vi "UHR-Fleezers Control (host) - Lorentz v5.vi"() -> ()   [LabVIEW 2014] (continued)
          n904 = property on="Invert laser interlacing" class="Bool (strict)"("Val(Sgnl)"=w1399) -> ()  [unwired: 2 in, 2 out]
          n905 = property on="Laser interlacing mode" class="RadioBtnsControl (strict)"("Val(Sgnl)"=w1400) -> ()  [unwired: 2 in, 2 out]
        }
        frame #2 {
          w1402 = path "C:/Home/Bustamante Lab/Comstock-LabView-Link.udl" ("connection information")
          # "Database link changed by Ronen - not clear if it matter for the program."
          # "Initialize the database connection"
          n906 = disable-structure shown="Disabled" {
            disable-tunnel: [w1405 _] -> w1403
            disable-tunnel: w1402 -> [w1404 _]
            frame Disabled {
              n907 = call-poly <vilib>:"DB Tools Open Connection.vi"("connection information"=w1404) -> ("connection reference"=w1405:T24)  [unwired: 7 in, 1 out]
            }
            frame Enabled {
            }
          }
          "connection reference" <- w1403
          n908 = local write "connection reference"(w1403) -> ()
          n909 = local write "Database link"(w1402) -> ()
        }
        frame #3 {
          # "Load active calibration to fpga"
          n910 = local read "Base N trap periods"() -> (w1407:u32)
          n911 = local read "T1 Osc Enable"() -> (w1406:bool)
          n912 = property on="T1 Osc Enable" class="Bool (strict)"("Val(Sgnl)"=w1406) -> ()  [unwired: 2 in, 2 out]
          n913 = property on="Base N trap periods" class="DigNum (strict)"("Val(Sgnl)"=w1407) -> ()  [unwired: 2 in, 2 out]
        }
      }
    }
    frame #4 {
      # "Set FIFO size and run FPGA"
      n914 = local read "FPGA error out"() -> (w1409:errorcluster)
      n915 = xnode "Invoke Method"("FPGA VI Reference In"=w1410, "error in"=w1409, "Requested Depth"="Trap AI FIFO Depth") -> ("FPGA VI Reference Out"=w1414:T35, "error out"=w1415:errorcluster)  [unwired: 1 out]
      n916 = xnode "Invoke Method"("FPGA VI Reference In"=w1414, "error in"=w1415, "Requested Depth"="Trap Position FIFO Depth") -> ("FPGA VI Reference Out"=w1412:T35, "error out"=w1411:errorcluster)  [unwired: 1 out]
      n917 = xnode "Invoke Method"("FPGA VI Reference In"=w1412, "error in"=w1411) -> ("error out"=w1408:errorcluster)  [unwired: 1 in, 1 out]
      n918 = local write "FPGA error out"(w1408) -> ()
    }
    frame #5 {
      # "Adjust FPGA timing loop phases"
      n919 = flat-sequence "Initial FPGA Loop Relative Phase Adjustment" {
        tunnel: "Initial Phase Adjustment (AI1)" -> [w1449]
        tunnel: "Initial Phase Adjustment (GI)" -> [w1448]
        tunnel: "Initial Phase Adj. (MCL)" -> [w1447]
        tunnel: [w1450] -> w1434
        tunnel: [w1446] -> w1433
        tunnel: "Initial Phase Adjustment (APD Acq)" -> [w1445]
        tunnel: "Initial Phase Adjustment (APD 1 Gate)" -> [w1444]
        tunnel: "Initial Phase Adjustment (Green FB)" -> [w1443]
        tunnel: "Initial Phase Adjustment (GI) 2" -> [w1442]
        tunnel: "Initial Phase Adjustment (APD 2 Gate)" -> [w1441]
        tunnel: "Initial Phase Adjustment (RI)" -> [w1440]
        tunnel: "Initial Phase Adjustment (BI DO)" -> [w1439]
        tunnel: "Initial Phase Adjustment (BI AO)" -> [w1438]
        tunnel: "Initial Phase Adjustment (APD 3 Gate)" -> [w1437]
        tunnel: w1419 -> [w1436]
        tunnel: w1434 -> [w1452]
        tunnel: [w1453] -> w1432
        tunnel: w1433 -> [w1453]
        tunnel: [w1452] -> w1431
        tunnel: w1432 -> [w1457]
        tunnel: w1431 -> [w1456]
        tunnel: [w1454] -> w1418
        frame #0 {
          n920 = local read "FPGA error out"() -> (w1435:errorcluster)
          n921 = xnode "Read/Write Control"("FPGA VI Reference In"=w1436, "error in"=w1435, "Phase count adjustment"=w1449, "Phase count adjustment (GI)"=w1448, "Phase count adjustment (MCL)"=w1447, "Phase Count Adjustment (APD Acq)"=w1445, "Phase count adjustment (APD 1 Gate)"=w1444, "Phase count adjustment (APD 2 Gate)"=w1441, "Phase count adjustment (Green FB)"=w1443, "Phase count adjustment (GI) 2"=w1442, "Phase count adjustment (RI)"=w1440, "Phase count adjustment (BI AO)"=w1438, "Phase count adjustment (BI D)"=w1439, "Phase count adjustment (APD 3 Gate)"=w1437) -> ("FPGA VI Reference Out"=w1446:T35, "error out"=w1450:errorcluster)
        }
        frame #1 {
          n922 = Wait (ms)(milliseconds to wait=u32 100) -> ()  [unwired: 1 out]
        }
        frame #2 {
          w1455 = TRUE
          n923 = xnode "Read/Write Control"("FPGA VI Reference In"=w1457, "error in"=w1456, "+ phase"=w1455, "+ phase (GI)"=w1455, "+ phase (MCL)"=w1455, "+ phase (APD Acq)"=w1455, "+ phase (APD 1 Gate)"=w1455, "+ phase (APD 2 Gate)"=w1455, "+ phase (Green FB)"=w1455, "+ phase (GI) 2"=w1455, "+ phase (RI)"=w1455, "+ phase (BI AO)"=w1455, "+ phase (BI D)"=w1455, "+ phase (APD 3 Gate)"=w1455) -> ("error out"=w1454:errorcluster)  [unwired: 1 out]
        }
      }
      n924 = local write "FPGA error out"(w1418) -> ()
    }
    frame #6 {
      w1471 = 6.0  # clock mult.
      w1470 = 49152000.0  # TCXO frequ.
      w1475 = 6.0  # clock mult.
      w1476 = 49152000.0  # TCXO frequ.
      # "Added by ronen - definition of \nlimit frequencies when using dynamic feedback"
      # "Initialize trap RF synth board and set initial frequencies and amplitudes"
      n925 = local read "FPGA error out"() -> (w1485:errorcluster)
      n926 = call "Initialize RF boards - interlace 3.vi"("error in"=w1485, "FPGA VI Reference In"=w1486) -> ("error out"=w1487:errorcluster, "FPGA VI Reference Out"=w1507:T35)
      n927 = call "set RF board frequency - interlace.vi"("Board 2 Frequency Limits"=w1482, "Board 1 Frequency Limits"=w1463, "error in"=w1487, "FPGA VI Reference In"=w1507, "Board 2 Frequency 3 (MHz)"="BD 2 Frequency 3 (MHz)", "Board 1 Frequency 3 (MHz)"="BD 1 Frequency 3 (MHz)", "Board 2 Frequency 2 (MHz)"="BD 2 Frequency 2 (MHz)", "Board 2 Frequency 1 (MHz)"="BD 2 Frequency 1 (MHz)", "Board 1 Frequency 2 (MHz)"="BD 1 Frequency 2 (MHz)", "Board 1 Frequency 1  (MHz)"="BD 1 Frequency 1 (MHz)") -> ("error out"=w1490:errorcluster, "FPGA VI Reference Out"=w1462:T35)
      n928 = Unbundle By Name(w1463) -> ("Maximum"=w1473:dbl, "Minimum"=w1464:dbl)
      n929 = call "set RF board amplitude - interlace.vi"("Board 2 Amplitude Limits"=w1484, "Board 1 Amplitude Limits"=w1483, "error in"=w1490, "FPGA VI Reference In"=w1462, "Board 2 Amplitude 3 (%)"="BD 2 Amplitude 3 (%)", "Board 1 Amplitude 3 (%)"="BD 1 Amplitude 3 (%)", "Board 2 Amplitude 2 (%)"="BD 2 Amplitude 2 (%)", "Board 2 Amplitude 1 (%)"="BD 2 Amplitude 1 (%)", "Board 1 Amplitude 2 (%)"="BD 1 Amplitude 2 (%)", "Board 1 Amplitude 1 (%)"="BD 1 Amplitude 1 (%)") -> ("error out"=w1459:errorcluster)  [unwired: 1 out]
      n930 = Multiply(x=w1464, y=1000000.0) -> (x*y=w1468:dbl)
      n931 = Multiply(x=w1473, y=1000000.0) -> (x*y=w1478:dbl)
      n932 = Scale By Power Of 2(n=48, x=w1468) -> (x*2^n=w1466:dbl)
      n933 = Subtract(x="BD 1 Frequency 1 (MHz)", y="BD 1 Frequency 2 (MHz)") -> (x-y=w1497:dbl)
      n934 = Subtract(x="BD 2 Frequency 1 (MHz)", y="BD 2 Frequency 2 (MHz)") -> (x-y=w1498:dbl)
      n935 = Scale By Power Of 2(n=48, x=w1478) -> (x*2^n=w1480:dbl)
      n936 = Multiply(x=w1470, y=w1471) -> (x*y=w1472:dbl)
      n937 = Multiply(x=w1476, y=w1475) -> (x*y=w1474:dbl)
      n938 = Square(x=w1498) -> (x^2=w1500:dbl)
      n939 = Square(x=w1497) -> (x^2=w1499:dbl)
      n940 = Divide(x=w1466, y=w1472) -> (x/y=w1467:dbl)
      n941 = Divide(x=w1480, y=w1474) -> (x/y=w1479:dbl)
      n942 = Add(x=w1499, y=w1500) -> (x+y=w1501:dbl)
      n943 = To Unsigned Quad Integer(1:w1467) -> (0:w1460:u64)
      n944 = To Unsigned Quad Integer(1:w1479) -> (0:w1461:u64)
      n945 = Square Root(x=w1501) -> (sqrt(x)=w1502:dbl)
      n946 = local write "Trap Delta (MHz)"(w1502) -> ()
      n947 = xnode "Read/Write Control"("FPGA VI Reference In"=w1462, "error in"=w1459, "FB Max Frequency"=w1461, "FB Min frequency"=w1460) -> ("error out"=w1458:errorcluster)  [unwired: 1 out]
      n948 = local write "FPGA error out"(w1458) -> ()
    }
    frame #7 {
      n949 = local read "FPGA error out"() -> (w1509:errorcluster)
      n950 = flat-sequence {
        tunnel: [w1523] -> w1514
        tunnel: [w1522] -> w1513
        tunnel: w1510 -> [w1516]
        tunnel: w1509 -> [w1515]
        tunnel: [w1527] -> w1512
        tunnel: w1514 -> [w1527]
        tunnel: [w1526] -> w1511
        tunnel: w1513 -> [w1526]
        tunnel: w1512 -> [w1535]
        tunnel: w1511 -> [w1534]
        tunnel: [w1529] -> w1508
        frame #0 {
          n951 = xnode "Read/Write Control"("FPGA VI Reference In"=w1516, "error in"=w1515, "Direct RF Box  Communication"=FALSE) -> ("FPGA VI Reference Out"=w1523:T35, "error out"=w1522:errorcluster)
          n952 = local read "Trap 1 (ON/OFF)"() -> (w1517:bool)
          n953 = local write "Saving..."(FALSE ("Saving Data")) -> ()
          n954 = local write "Stop All"(FALSE ("Stop All")) -> ()
          n955 = local write "Index"(1.0 ("Index")) -> ()
          n956 = property on="Trap 1 ON" class="Bool (strict)"("Value"=w1517) -> ()  [unwired: 2 in, 2 out]
          "Manipulating Trap" <- FALSE ("Manipulating Trap")
        }
        frame #1 {
          n957 = local read "Trap 2 (ON/OFF)"() -> (w1525:bool)
          n958 = Wait (ms)(milliseconds to wait=u32 10) -> ()  [unwired: 1 out]
          n959 = property on="Trap 2 ON" class="Bool (strict)"("Val(Sgnl)"=w1525) -> ()  [unwired: 2 in, 2 out]
        }
        frame #2 {
          n960 = local read "Scan Range (nm)"() -> (w1530:dbl)
          n961 = xnode "Read/Write Control"("FPGA VI Reference In"=w1535, "error in"=w1534, "FPGA Controls  RF Box"=TRUE ("Direct RF Box  Communication")) -> ("error out"=w1529:errorcluster)  [unwired: 1 out]
          n962 = call "Update messages.vi"("Message to add"="UHR-Fleezers ready.", "Old message string"="") -> ("New message string"=w1533:string)
          n963 = local write "Messages"(w1533) -> ()
          n964 = property on="Scan Range (nm)" class="DigNum (strict)"("Val(Sgnl)"=w1530) -> ()  [unwired: 2 in, 2 out]
        }
      }
      n965 = local write "FPGA error out"(w1508) -> ()
    }
    frame #8 {
      w1542 = u32 0
      w1548 = cluster{u32, u32} {16777238, 16777238}
      w1543 = 0.0
      n966 = control-ref of="Piezo trap cursor control"() -> (w1544:refnum<vi>)
      n967 = property class="XYGraph (strict)"(reference=w1544, "XScale.Maximum"=10.0, "XScale.Minimum"=w1543, "YScale.Maximum"=w1543, "YScale.Minimum"=-10.0, "Plot Area Colors"=w1548, "Frame Color"=u32 9868950, "XScale.GridColors"=w1548, "YScale.GridColors"=w1548, "Cursor.Cursor Color"=u32 16711680, "Active Cursor"=w1542, "Cursor.CursorMode"=w1542) -> ()  [unwired: 1 in, 2 out]
      n968 = call "hamilton_controller.vi"("VISA resource name in"="Visa resource for valves", "action"=T41."CONNECT") -> ("error out"=w1541:errorcluster, "VISA resource name out"=w1538:refnum<visa-resource-name>)  [unwired: 8 in]
      n969 = call "hamilton_controller.vi"("VISA resource name in"=w1538, "error in"=w1541, "action"=T41."INITIALIZE VALVES") -> ("error out"=w1550:errorcluster)  [unwired: 7 in, 1 out]
    }
    frame #9 {
      # "Wait 5 s for all the event loops still being executed to finish."
      n970 = Wait (ms)(milliseconds to wait=u32 5000) -> ()  [unwired: 1 out]
      n971 = local read "FPGA error out"() -> (w1552:errorcluster)
    }
  }
  n972 = node-c288() -> (w30:T36)  [unwired: 4 out]
  n973 = disable-structure shown="Disabled" {
    frame Disabled {
      n974 = while "Duncan's play event loop" {
        stop <- w1556 stop-if-true
        n975 = Create User Event(user event datatype=TRUE ("Boolean")) -> (user event=w1557:refnum<user-event>)  [unwired: 1 in, 1 out]
        n976 = Create User Event(user event datatype=TRUE ("Boolean")) -> (user event=w1563:refnum<user-event>)  [unwired: 1 in, 1 out]
        n977 = global write "Global for fluorescence simulation mean (30 samples), (power series).vi" "Red Signal"(w1557) -> ()
        n978 = global write "Global for fluorescence simulation mean (30 samples), (power series).vi" "Green Signal"(w1563) -> ()
        n979 = register-events(w1563, w1557) -> (reference out=w1562:refnum<event-registration>)  [unwired: 2 in, 1 out]
        n980 = event shown="[1] \"Start assembly line\": Value Change" {
          selector: w1562 -> [_ _ _ _]
          dyn-events: _ -> [_ _ _ _]
          timeout: 100 -> [_ _ _ _]
          event Timeout {
            n981 = event-data() -> ()  [unwired: 1 in, 2 out]
          }
          event "Start assembly line": Value Change {
            n982 = event-data() -> ("OldVal"=w1565:bool)  [unwired: 1 in, 4 out]
            n983 = case shown="True" w1565 {
              selector: w1565 -> [_ w1566]
              frame False {
              }
              frame True {
                n984 = property on="Move to Position 3" class="Bool"("Val(Sgnl)"=w1566) -> ()  [unwired: 2 in, 2 out]
                n985 = case shown="1" "Numeric" {
                  frame 0, Default {
                  }
                  frame 1 {
                    n986 = property on="Green Laser ON" class="Bool (strict)"("Val(Sgnl)"=TRUE ("Value (Signaling)")) -> ()  [unwired: 2 in, 2 out]
                  }
                  frame 2 {
                    n987 = property on="Red Laser ON" class="Bool (strict)"("Val(Sgnl)"=TRUE) -> ()  [unwired: 2 in, 2 out]
                  }
                }
              }
            }
          }
          event User Event {
            n988 = event-data() -> ("Boolean"=w1570:bool)  [unwired: 1 in, 3 out]
            "Green Fluorophore" <- w1570
            n989 = property on="Start assembly line" class="Bool"("Val(Sgnl)"=w1570) -> ()  [unwired: 2 in, 2 out]
          }
          event User Event {
            n990 = event-data() -> ("Boolean"=w1571:bool)  [unwired: 1 in, 3 out]
            "Red Fluorophore" <- w1571
            n991 = property on="Start assembly line" class="Bool"("Val(Sgnl)"=w1571) -> ()  [unwired: 2 in, 2 out]
          }
        }
        n992 = property on="Get Fluorophore" class="Bool (strict)"("Val(Sgnl)"="Get Fluorophore") -> ()  [unwired: 2 in, 2 out]
        n993 = Wait (ms)(milliseconds to wait=u32 100) -> ()  [unwired: 1 out]
        n994 = local read "Stop All"() -> (w1555:bool)
        n995 = Or(x=w1555, y="stop") -> (x .or. y?=w1556:bool)
      }
    }
    frame Enabled {
    }
  }
  n996 = timed-loop "Rough control of MCL mirror stage (debugging)" {
    tunnel: [w1574] -> w71
    timing: w30 -> [_]
    timing-out: [_] -> w29
    tunnel: w21 -> [w1572]
    stop <- w1574 stop-if-true
    n997 = node-c288() -> ()  [unwired: 2 out]
    n998 = case shown="1" "MCL Mode" {
      tunnel: w1572 -> [_ w1577 w1624]
      frame 0, Default {
      }
      frame 1 {
        n999 = node-c288() -> (w1579:T36)  [unwired: 4 out]
        n1000 = timed-loop "Oscillate MCL mirror" {
          timing: w1579 -> [_]
          timing-out: [_] -> w1578
          tunnel: w1577 -> [w1580]
          i -> [w1618]
          stop <- w1581 stop-if-true
          n1001 = node-c288() -> (w1617:i64)  [unwired: 1 out]
          n1002 = Multiply(x="AO1", y=32767.0) -> (x*y=w1613:dbl)
          n1003 = Multiply(x="AO2", y=32767.0) -> (x*y=w1608:dbl)
          n1004 = Divide(x=w1613, y=10.0) -> (x/y=w1614:dbl)
          n1005 = Divide(x=w1608, y=10.0) -> (x/y=w1609:dbl)
          n1006 = To Word Integer(number=w1614) -> (16bit integer=w1606:i16)
          n1007 = To Word Integer(number=w1609) -> (16bit integer=w1605:i16)
          n1008 = Divide(x=w1617, y=i64 1000) -> (x/y=w1588:dbl)
          n1009 = Multiply(x=w1588, y=w1618) -> (x*y=w1599:dbl)
          n1010 = Multiply(x="Osc. freq. (Hz) 2", y=6.283185307179586) -> (x*y=w1600:dbl)
          n1011 = Multiply(x=w1600, y=w1599) -> (x*y=w1598:dbl)
          n1012 = Sine(x=w1598) -> (sin(x)=w1597:dbl)
          n1013 = Multiply(x=w1597, y="Osc. amp. (V)") -> (x*y=w1595:dbl)
          n1014 = Add(x=w1595, y="Osc. center (V)") -> (x+y=w1593:dbl)
          n1015 = Divide(x=w1593, y=10.0) -> (x/y=w1591:dbl)
          n1016 = Multiply(x=w1591, y=32767.0) -> (x*y=w1586:dbl)
          n1017 = Select(t=w1586, s="Scan axis", f=w1606) -> (s? t:f=w1604:dbl)
          n1018 = Select(t=w1605, s="Scan axis", f=w1586) -> (s? t:f=w1603:dbl)
          n1019 = local read "MCL Mode"() -> (w1585:u16)
          n1020 = Not Equal?(x=w1585, y=u16 1) -> (x != y?=w1582:bool)
          n1021 = local read "Stop All"() -> (w1583:bool)
          n1022 = xnode "Read/Write Control"("FPGA VI Reference In"=w1580, "AO1"=w1604, "AO2"=w1603) -> ()  [unwired: 1 in, 2 out]
          n1023 = Compound Arithmetic op=OR(w1583, w1582) -> (w1581:bool)
          n1024 = node-c288() -> ()  [unwired: 2 out]
        }
        n1025 = node-c288(w1578) -> ()  [unwired: 1 out]
      }
      frame 2 {
        n1026 = case shown="True" "Start Scan" {
          tunnel: w1624 -> [_ w1626]
          frame False {
          }
          frame True {
            n1027 = Subtract(x="End (V)", y="Begin (V)") -> (x-y=w1633:dbl)
            n1028 = Decrement(x="N Points") -> (x-1=w1632:dbl)
            n1029 = Divide(x=w1633, y=w1632) -> (x/y=w1630:dbl)
            n1030 = for {
              N: "N Points" -> [_]
              tunnel: "Begin (V)" -> [w1649]
              tunnel: [w1641] -> w1636 mode=indexing
              tunnel: w1630 -> [w1640]
              tunnel: [w1638] -> w1629 mode=indexing
              tunnel: w1626 -> [w1637]
              i -> [w1648]
              n1031 = Multiply(x=w1640, y=w1648) -> (x*y=w1647:dbl)
              n1032 = Add(x=w1649, y=w1647) -> (x+y=w1644:dbl)
              n1033 = local read "Scan axis"() -> (w1639:bool)
              n1034 = local read "AO1"() -> (w1646:dbl)
              n1035 = local read "AO2"() -> (w1645:dbl)
              n1036 = Select(t=w1644, s=w1639, f=w1646) -> (s? t:f=w1643:dbl)
              n1037 = Select(t=w1645, s=w1639, f=w1644) -> (s? t:f=w1642:dbl)
              n1038 = flat-sequence {
                tunnel: w1643 -> [w1653]
                tunnel: w1642 -> [w1652]
                tunnel: w1637 -> [w1650]
                tunnel: [w1663] -> w1641
                tunnel: [w1662] -> w1638
                frame #0 {
                  w1656 = 10.0 ("y")
                  w1651 = 32767.0 ("y")
                  n1039 = Multiply(x=w1653, y=w1651) -> (x*y=w1659:dbl)
                  n1040 = Multiply(x=w1652, y=w1651) -> (x*y=w1657:dbl)
                  n1041 = Divide(x=w1659, y=w1656) -> (x/y=w1660:dbl)
                  n1042 = Divide(x=w1657, y=w1656) -> (x/y=w1658:dbl)
                  n1043 = To Word Integer(number=w1660) -> (16bit integer=w1654:i16)
                  n1044 = To Word Integer(number=w1658) -> (16bit integer=w1655:i16)
                  n1045 = xnode "Read/Write Control"("FPGA VI Reference In"=w1650, "AO1"=w1654, "AO2"=w1655) -> ()  [unwired: 1 in, 2 out]
                }
                frame #1 {
                  n1046 = Wait (ms)(milliseconds to wait="DAQ Delay (ms)") -> ()  [unwired: 1 out]
                }
                frame #2 {
                  n1047 = local read "Slow mean"() -> (w1663:dbl)
                  n1048 = local read "Sigma"() -> (w1662:dbl)
                }
              }
            }
            n1049 = Bundle("Begin (V)"="Begin (V)", w1630, w1636) -> (→"MCL Scan":cluster{"Begin (V)":dbl, dbl, dbl[]})  [unwired: 1 out]
            n1050 = Bundle("Begin (V)"="Begin (V)", w1630, w1629) -> (→"MCL Scan 2":cluster{"Begin (V)":dbl, dbl, dbl[]})  [unwired: 1 out]
          }
        }
      }
    }
    n1051 = local read "Stop All"() -> (w1574:bool)
    n1052 = node-c288() -> ()  [unwired: 2 out]
  }
  n1053 = node-c288(2 ("Processor")) -> (w62:T36)  [unwired: 3 out]
  n1054 = timed-loop "Basic control parameters (all FPGA settings, other basic controls)" {
    shift-right: [w1671] -> _
    shift-left: errorcluster {"status"=FALSE, "code"=0, "source"=""} ("error out") -> [_]
    tunnel: [w1670] -> _
    timing: w62 -> [_]
    timing-out: [_] -> w61
    tunnel: w43 -> [w1669]
    tunnel: w39 -> [w1668]
    tunnel: w38 -> [w1667]
    tunnel: w37 -> [w1666]
    tunnel: w36 -> [w1665]
    tunnel: w21 -> [w1664]
    stop <- w1670 stop-if-true
    n1055 = node-c288() -> ()  [unwired: 2 out]
    n1056 = event shown="[0] \"AI Count (ticks)\", \"Sets to FIFO (Traps)\", \"Save ave N\", \"FPGA Ave.\", \"# Samples/channel\", \"N sets to save\": Value Change" {
      selector: _ -> [_ _ _ _ _ _ _ _ _ _ _ _ _ _ _ _ _ _ _ _ _ _ _ _ _ _ _ _ _ _ _ _ _ _ _ _ _ _ _ _ _ _ _ _ _ _ _ _ _ _ _ _ _ _ _ _ _ _ _ _ _ _ _ _ _ _ _ _ _ _ _ _ _ _ _ _ _ _ _ _ _ _ _ _ _ _]
      dyn-events: _ -> [_ _ _ _ _ _ _ _ _ _ _ _ _ _ _ _ _ _ _ _ _ _ _ _ _ _ _ _ _ _ _ _ _ _ _ _ _ _ _ _ _ _ _ _ _ _ _ _ _ _ _ _ _ _ _ _ _ _ _ _ _ _ _ _ _ _ _ _ _ _ _ _ _ _ _ _ _ _ _ _ _ _ _ _ _ _]
      timeout: _ -> [_ _ _ _ _ _ _ _ _ _ _ _ _ _ _ _ _ _ _ _ _ _ _ _ _ _ _ _ _ _ _ _ _ _ _ _ _ _ _ _ _ _ _ _ _ _ _ _ _ _ _ _ _ _ _ _ _ _ _ _ _ _ _ _ _ _ _ _ _ _ _ _ _ _ _ _ _ _ _ _ _ _ _ _ _ _]
      tunnel: [w1711 _ _ _ w1738 _ _ _ _ _ _ _ w1844 _ _ w1931 w1933 w1940 w1942 w2012 _ w2054 w2080 w2108 w2133 w2160 w2186 w2215 _ w2220 w2314 w2318 w2355 _ w2418 w2421 w2424 w2434 w2437 _ w2444 _ _ _ _ _ _ _ _ _ _ _ _ _ _ _ _ _ _ _ w2939 _ _ _ _ w2976 _ _ _ _ _ _ _ _ _ _ _ _ _ _ _ _ _ _ _ _] -> w1671
      tunnel: [_ _ _ _ _ _ _ _ _ _ w1823 _ _ _ _ _ _ _ _ _ _ _ _ _ _ _ _ _ _ _ _ _ _ _ _ _ _ _ _ _ _ _ _ _ _ _ _ _ _ _ _ _ _ _ _ _ _ _ _ _ _ _ _ _ _ _ _ _ _ _ _ _ _ _ _ _ _ _ _ _ _ _ _ _ _ _] -> w1670
      tunnel: [_ _ _ _ _ _ _ _ "Round T1 X" _ _ _ _ _ _ _ _ _ _ _ _ _ _ _ _ _ _ _ _ _ _ _ _ _ _ _ _ _ _ _ _ _ _ _ _ _ _ _ _ _ _ _ _ _ _ _ _ _ _ _ _ _ _ _ _ _ _ _ _ _ _ _ _ _ _ _ _ _ _ _ _ _ _ _ _ _] -> _
      tunnel: [_ _ _ "Adjust Scale\nto Mean" _ _ _ _ _ _ _ _ _ _ _ _ _ _ _ _ _ _ _ _ _ _ _ _ _ "Test ttrig" _ _ _ _ _ _ _ _ _ _ _ _ _ _ _ _ _ _ _ _ w2686 w2750 w2797 w2846 _ _ _ _ _ _ _ _ _ _ _ _ _ _ _ _ _ _ _ _ _ _ _ _ _ _ _ _ _ _ _ _] -> _
      tunnel: [_ _ _ _ _ _ _ _ _ "Round T2 X" _ "Delayed Interlace Start" _ _ _ _ _ _ _ _ _ _ _ _ _ _ _ _ _ _ _ _ _ _ _ _ _ _ _ _ _ _ _ _ _ _ _ _ _ _ _ _ _ _ _ _ _ _ _ _ _ _ _ _ _ _ _ _ _ _ _ _ _ _ _ _ _ _ _ _ _ _ _ _ _ _] -> _
      tunnel: w1669 -> [_ _ _ _ _ _ _ _ _ _ _ _ _ _ _ _ _ _ _ _ _ _ _ _ _ _ _ _ _ _ _ _ _ _ _ _ _ _ _ _ _ _ _ _ _ _ w2656 w2664 w2671 w2677 w2685 _ _ w2845 _ _ _ _ _ _ _ _ _ _ _ _ _ _ _ _ _ _ _ _ _ _ _ _ _ _ _ _ _ _ _ _]
      tunnel: w1668 -> [_ _ _ _ _ _ _ _ _ _ _ _ _ _ _ _ _ _ _ _ _ _ _ _ _ _ _ _ _ _ _ _ _ _ _ _ _ _ _ _ _ _ _ _ w2543 _ _ _ _ _ _ w2749 _ _ w2852 _ w2864 _ w2880 _ _ _ _ _ _ _ _ _ _ _ _ _ _ _ _ _ _ _ _ _ _ _ _ _ _ _]
      tunnel: w1667 -> [_ _ _ _ _ _ _ _ _ _ _ _ _ _ _ _ _ _ _ _ _ _ _ _ _ _ _ _ _ _ _ _ _ _ _ _ _ _ _ _ _ _ _ _ _ _ _ _ _ _ _ _ _ _ _ _ _ _ _ _ _ _ _ _ _ _ _ _ _ _ _ _ _ _ _ _ _ _ _ _ _ _ _ _ _ _]
      tunnel: w1666 -> [_ _ _ _ _ _ _ _ _ _ _ _ _ _ _ _ _ _ _ _ _ _ _ _ _ _ _ _ _ _ _ _ _ _ _ _ _ _ _ _ _ w2455 _ _ _ _ _ _ _ _ _ _ w2796 _ _ w2858 _ w2872 _ w2906 _ _ _ _ _ _ _ _ _ _ _ _ _ _ _ _ _ _ _ _ _ _ _ _ _ _]
      tunnel: w1665 -> [_ _ _ _ _ _ _ _ _ _ _ _ _ _ _ _ _ _ _ _ _ _ _ _ _ _ _ _ _ _ _ _ _ _ _ _ _ _ _ _ _ _ _ _ _ _ _ _ _ _ _ _ _ _ _ _ _ _ _ _ _ _ _ _ _ _ _ _ _ _ _ _ _ _ _ _ _ _ _ _ _ _ _ _ _ _]
      tunnel: w1664 -> [w1674 _ _ _ w1737 _ w1763 _ _ _ _ _ w1835 _ _ w1915 w1932 w1939 w1941 w1977 _ w2043 w2078 w2090 w2115 w2143 w2163 w2191 w2216 w2218 w2222 w2315 w2319 _ w2415 w2419 w2422 w2432 w2435 _ w2443 _ _ _ _ _ _ _ _ _ _ _ _ _ _ _ _ _ _ _ w2932 _ w2953 _ w2960 w2975 _ w2982 w3009 w3016 w3032 w3040 _ w3051 _ w3095 _ _ w3149 w3180 w3184 w3192 _ w3256 w3266 w3285]
      tunnel: [_ _ _ _ _ _ _ _ _ _ w1822 _ _ _ _ _ _ _ _ _ _ _ _ _ _ _ _ _ _ _ _ _ _ _ _ _ _ _ _ _ _ _ w2535 w2539 _ _ _ _ _ _ _ _ _ _ _ _ _ _ _ _ _ _ _ _ _ _ _ _ _ _ _ _ _ _ _ _ _ _ _ _ _ _ _ _ _ _] -> _
      event "AI Count (ticks)", "Sets to FIFO (Traps)", "Save ave N", "FPGA Ave.", "# Samples/channel", "N sets to save": Value Change {
        # "RG 18-01-16 Increased amount of elements to read for trap position, to add x and y for piezo trap"
        # "So that if 'Save ave N' is updated, the AOD scanning code updates too."
        n1057 = event-data() -> ()  [unwired: 6 out]
        n1058 = local read "AI Count (ticks)"() -> (w1695:u16)
        n1059 = Divide(x=40000000.0, y=w1695) -> (x/y=w1687:dbl)
        "AI rate (Hz)" <- w1687
        "Ave. Rate (Hz)" <- w1687
        n1060 = Reciprocal(x=w1687) -> (1/x=→"Ave. Period (s)":dbl)
        n1061 = Unbundle By Name("Sets to FIFO (Traps)") -> ("Set 1"=w1678:bool, "Set 2"=w1677:bool, "Set 3"=w1676:bool)
        n1062 = Divide(x=w1687, y="N Acq Sets (Traps + Fl.)") -> (x/y=w1708:dbl)
        "Data Rate (Hz)" <- w1708
        n1063 = Reciprocal(x=w1708) -> (1/x=→"Data Period (s)":dbl)
        n1064 = Boolean To (0,1)(Boolean="Sets to FIFO (Traps)") -> (0, 1=w1703:cluster{"Set 1":i16, "Set 2":i16, "Set 3":i16})
        n1065 = xnode "Read/Write Control"("FPGA VI Reference In"=w1674, "ai count"=w1695, "Set 1"=w1678, "Set 2"=w1677, "Set 3"=w1676, "N of AI1 Int Acq Sets"="N Acq Sets (Traps + Fl.)") -> ("error out"=w1711:errorcluster)  [unwired: 1 in, 1 out]
        n1066 = Cluster To Array(cluster=w1703) -> (array=w1702:i16[])
        n1067 = local read "Save ave N"() -> (w1707:dbl)
        n1068 = To Unsigned Long Integer(number=w1702) -> (unsigned 32bit integer=w1684:u32[])
        n1069 = local read "Scan steps (AOD)"() -> (w1704:u64)
        n1070 = Multiply(x=w1695, y="N Acq Sets (Traps + Fl.)") -> (x*y=w1693:u16)
        n1071 = Add Array Elements(numeric array=w1684) -> (sum=w1696:u32)
        "Trap Sets" <- w1696
        n1072 = Divide(x=w1708, y=w1707) -> (x/y=w1706:dbl)
        "Save Data Rate (Hz)" <- w1706
        n1073 = Reciprocal(x=w1706) -> (1/x=→"Save Data Period (s)":dbl)
        n1074 = property on="Scan steps (AOD)" class="DigNum (strict)"("Val(Sgnl)"=w1704) -> ()  [unwired: 2 in, 2 out]
        n1075 = Multiply(x=w1693, y="# Samples/trap") -> (x*y=w1691:u32)
        "Counts/DMA" <- w1691
        n1076 = property on="Trap Disp. Downsample" class="DigNum (strict)"("Maximum"="# Samples/trap") -> ()  [unwired: 2 in, 2 out]
        n1077 = Multiply(x=w1696, y="# Samples/trap") -> (x*y=w1685:u32)
        "# Samples/channel" <- w1685
        n1078 = Multiply(x=w1685, y=u32 8) -> (x*y=→"Trap AI Elements/DMA read":u32)
        n1079 = local read "APD Int. Count"() -> (w1692:u32)
        n1080 = Multiply(x=w1685, y=u32 5) -> (x*y=→"Trap Pos Elements/DMA read":u32)
        n1081 = Divide(x=w1691, y=w1692) -> (x/y=w1682:dbl)
        "APD Samples/FIFO Acq." <- w1682
        n1082 = Divide(x=w1691, y=40000000.0) -> (x/y=w1689:dbl)
        "DMA Update Period (s)" <- w1689
        n1083 = local read "Number of APDs"() -> (w1675:u8)
        n1084 = Multiply(x=w1675, y=w1682) -> (x*y=→"APD Elements/DMA read":dbl)
        n1085 = property on="APD Disp. Downsample" class="DigNum (strict)"("Maximum"=w1682) -> ()  [unwired: 2 in, 2 out]
        n1086 = local read "N sets to save"() -> (w1701:u32)
        n1087 = Multiply(x=w1689, y=w1701) -> (x*y=→"Total Time (s) 2":dbl)
        "FPGA Averaging" <- FALSE ("FPGA Averaging")
      }
      event "Remove Offset": Value Change {
        n1088 = event-data() -> ()  [unwired: 7 out]
        n1089 = local write "Remove Offset"(FALSE ("Remove Offset")) -> ()
        n1090 = local read "Bead Mean (nm)"() -> (w1713:dbl)
        n1091 = local read "Offset (nm)"() -> (w1714:dbl)
        n1092 = Add(x=w1713, y=w1714) -> (x+y=w1712:dbl)
        n1093 = local write "Offset (nm)"(w1712) -> ()
      }
      event "Detector Type": Value Change {
        n1094 = event-data() -> ()  [unwired: 7 out]
        n1095 = local read "AI labels"() -> (w1718:string[])
        n1096 = property on="High Res. Display" class="Ring (strict)"("Strings []"=w1718) -> ()  [unwired: 2 in, 2 out]
        n1097 = Build Array (concatenate)(w1718, "none") -> (w1719:string[])
        n1098 = property on="FFT 1 Choice 1" class="Ring (strict)"("Strings []"=w1719) -> ()  [unwired: 2 in, 2 out]
        n1099 = property on="FFT 1 Choice 2" class="Ring (strict)"("Strings []"=w1719) -> ()  [unwired: 2 in, 2 out]
        n1100 = property on="FFT 2 Choice 1" class="Ring (strict)"("Strings []"=w1719) -> ()  [unwired: 2 in, 2 out]
        n1101 = property on="FFT 2 Choice 2" class="Ring (strict)"("Strings []"=w1719) -> ()  [unwired: 2 in, 2 out]
        n1102 = Bundle("APD 1", "APD 2", "APD 3") -> (w1722:cluster{string, string, string})  [unwired: 1 out]
        n1103 = Cluster To Array(cluster=w1722) -> (array=w1720:string[])
        n1104 = Build Array (concatenate)(w1720, w1719) -> (w1724:string[])
        n1105 = Array Size(array=w1724) -> (size(s)=w1716:i32)
        n1106 = property on="Signals to Plot" class="LstBox (strict)"("Item Names"=w1724) -> ()  [unwired: 2 in, 2 out]
        n1107 = property on="Signals to Plot" class="LstBox (strict)"("Number of Rows"=w1716) -> ()  [unwired: 2 in, 2 out]
        n1108 = property on="All Signals" class="WFChart (strict)"("LegNumRows"=w1716) -> ()  [unwired: 2 in, 2 out]
      }
      event "Adjust Scale\nto Mean": Value Change {
        n1109 = event-data() -> ()  [unwired: 7 out]
        n1110 = local read "APD rates cluster"() -> (w1727:T1)
        n1111 = Unbundle By Name(w1727) -> ("APD 1 Rate (Hz)"=w1726:dbl)
        n1112 = Multiply(x=1000.0, y="Above (kHz)") -> (x*y=w1733:dbl)
        n1113 = Multiply(x=1000.0, y="Below (kHz)") -> (x*y=w1731:dbl)
        n1114 = Add(x=w1733, y=w1726) -> (x+y=w1728:dbl)
        n1115 = Subtract(x=w1726, y=w1731) -> (x-y=w1729:dbl)
        n1116 = property on="APD Chart" class="WFChart (strict)"("YScale.Minimum"=w1729) -> ()  [unwired: 2 in, 2 out]
        n1117 = property on="APD Chart" class="WFChart (strict)"("YScale.Maximum"=w1728) -> ()  [unwired: 2 in, 2 out]
      }
      event "Phase adj. (AI1)", "+ phase (AI1)", "- phase (AI1)": Value Change {
        n1118 = event-data() -> ()  [unwired: 7 out]
        n1119 = Negate(x="Phase adj. (AI1)") -> (-x=w1745:i16)
        n1120 = Select(t=w1745, s="- phase (AI1)", f="Phase adj. (AI1)") -> (s? t:f=w1744:i16)
        n1121 = xnode "Read/Write Control"("FPGA VI Reference In"=w1737, "Phase count adjustment"=w1744) -> ("FPGA VI Reference Out"=w1743:T35, "error out"=w1742:errorcluster)  [unwired: 2 in]
        n1122 = Or(x="- phase (AI1)", y="+ phase (AI1)") -> (x .or. y?=w1739:bool)
        n1123 = xnode "Read/Write Control"("FPGA VI Reference In"=w1743, "error in"=w1742, "+ phase"=w1739) -> ("error out"=w1738:errorcluster)  [unwired: 1 in, 1 out]
      }
      event "Signals to Plot": Double Click {
        w1757 = u32 9868950 ("Color Box")
        n1124 = event-data() -> ("Row"=w1748:i32)  [unwired: 9 out]
        n1125 = property on="All Signals" class="WFChart (strict)"("Active Plot"=w1748) -> (error out=w1747:errorcluster)  [unwired: 2 in, 1 out]
        n1126 = property on="All Signals" class="WFChart (strict)" props=["Plot", "Plot Color", "Plot", "Visible?"](error in=w1747) -> (error out=w1750:errorcluster, "Plot.Visible?"=w1749:bool)  [unwired: 1 in, 2 out]
        n1127 = Select(t=FALSE ("Plot.Visible"), s=w1749, f=TRUE ("Plot.Visible")) -> (s? t:f=w1752:bool)
        n1128 = property on="All Signals" class="WFChart (strict)"(error in=w1750, "Plot.Visible?"=w1752) -> (error out=w1751:errorcluster)  [unwired: 1 in, 1 out]
        n1129 = property on="All Signals" class="WFChart (strict)"(error in=w1751) -> (error out=w1753:errorcluster, "Plot.Plot Color"=w1754:u32)  [unwired: 1 in, 1 out]
        n1130 = property on="Signals to Plot" class="LstBox (strict)"(error in=w1753, "Active Row"=w1748) -> (error out=w1758:errorcluster)  [unwired: 1 in, 1 out]
        n1131 = Select(t=w1754, s=w1752, f=u32 0) -> (s? t:f=w1759:u32)
        n1132 = property on="Signals to Plot" class="LstBox (strict)"(error in=w1758, "CellFontColor"=w1759, "SelColor"=w1757, "CellBG"=w1757, "CellFontSize"=u32 20 ("Active Row:Cell Font:Size"), "CellFontBold"=TRUE ("Active Row:Cell Font:Bold")) -> ()  [unwired: 1 in, 2 out]
      }
      event "BD 1 Frequency 1 (MHz)", "BD 1 Frequency 2 (MHz)", "BD 1 Frequency 3 (MHz)", "BD 2 Frequency 1 (MHz)", "BD 2 Frequency 2 (MHz)", "BD 2 Frequency 3 (MHz)", "Trap Delta (MHz)", "Update all trap values": Value Change {
        # "This is so you can set trap frequencies\nvia local variables and then update\nall at once"
        n1133 = event-data() -> ("CtlRef"=w1767:refnum<vi>)  [unwired: 6 out]
        n1134 = control-ref of="Trap Delta (MHz)"() -> (w1766:refnum<vi>)
        n1135 = Equal?(x=w1766, y=w1767) -> (x = y?=w1765:bool)
        n1136 = local write "Update all trap values"(FALSE ("Update all trap values")) -> ()
        n1137 = case shown="False" "Oscillate Set 1" {
          tunnel: w1765 -> [w1781 _]
          tunnel: w1763 -> [w1779 _]
          frame False {
            n1138 = local read "BD 1 Frequency 2 (MHz)"() -> (w1777:dbl)
            n1139 = case shown="False" "Symmetric?" {
              tunnel: "Trap Delta (MHz)" -> [w1803 w1810]
              tunnel: [w1804 w1808] -> w1769
              tunnel: [w1802 w1805] -> w1771
              tunnel: w1777 -> [w1804 _]
              frame False {
                n1140 = Subtract(x=w1804, y=w1803) -> (x-y=w1802:dbl)
              }
              frame True {
                w1807 = 75
                n1141 = Divide(x=w1810, y=2.0) -> (x/y=w1806:dbl)
                n1142 = Add(x=w1806, y=w1807) -> (x+y=w1808:dbl)
                n1143 = Subtract(x=w1807, y=w1806) -> (x-y=w1805:dbl)
              }
            }
            n1144 = local read "BD 1 Frequency 1 (MHz)"() -> (w1772:dbl)
            n1145 = Not(x="Symmetric?") -> (.not. x?=w1775:bool)
            n1146 = And(x=w1775, y="move Con X?") -> (x .and. y?=w1773:bool)
            n1147 = Subtract(x=w1772, y=w1771) -> (x-y=w1770:dbl)
            n1148 = Select(t=w1771, s=w1781, f=w1772) -> (s? t:f=w1780:dbl)
            n1149 = local read "Y RF Frequency Limits (MHz)"() -> (w1782:T23)
            n1150 = case shown="True" w1773 {
              tunnel: w1770 -> [_ w1801]
              frame False {
              }
              frame True {
                n1151 = property on="AOM X Cal (nm/MHz)" class="DigNum (strict)"() -> ("Value"=w1800:dbl)  [unwired: 2 in, 2 out]
                n1152 = property on="MCL Step Position Ratio" class="DigNum (strict)"() -> ("Value"=w1794:dbl)  [unwired: 2 in, 2 out]
                n1153 = Compound Arithmetic op=MULTIPLY(w1801, w1800, w1794) -> (w1799:dbl)
                n1154 = property on="MCL X Cal (nm/V)" class="DigNum (strict)"() -> ("Value"=w1798:dbl)  [unwired: 2 in, 2 out]
                n1155 = Divide(x=w1799, y=w1798) -> (x/y=w1797:dbl)
                n1156 = property on="AO2" class="Slide (strict)"() -> ("Value"=w1796:dbl)  [unwired: 2 in, 2 out]
                n1157 = Add(x=w1797, y=w1796) -> (x+y=w1795:dbl)
                n1158 = property on="AO2" class="Slide (strict)"("Val(Sgnl)"=w1795) -> ()  [unwired: 2 in, 2 out]
              }
            }
            n1159 = local read "X RF Frequency Limits (MHz)"() -> (w1783:T23)
            n1160 = local write "BD 1 Frequency 1 (MHz)"(w1780) -> ()
            n1161 = local read "BD 1 Frequency 3 (MHz)"() -> (w1792:dbl)
            n1162 = local read "BD 2 Frequency 1 (MHz)"() -> (w1786:dbl)
            n1163 = local read "BD 2 Frequency 2 (MHz)"() -> (w1785:dbl)
            n1164 = local read "BD 2 Frequency 3 (MHz)"() -> (w1793:dbl)
            n1165 = call "set RF board frequency - interlace.vi"("Board 2 Frequency Limits"=w1782, "Board 1 Frequency Limits"=w1783, "FPGA VI Reference In"=w1779, "Board 2 Frequency 3 (MHz)"=w1793, "Board 1 Frequency 3 (MHz)"=w1792, "Board 2 Frequency 2 (MHz)"=w1785, "Board 2 Frequency 1 (MHz)"=w1786, "Board 1 Frequency 2 (MHz)"=w1769, "Board 1 Frequency 1  (MHz)"=w1780) -> ()  [unwired: 1 in, 2 out]
            n1166 = Subtract(x=w1786, y=w1785) -> (x-y=w1790:dbl)
            n1167 = local write "BD 1 Frequency 2 (MHz)"(w1769) -> ()
            n1168 = Subtract(x=w1780, y=w1769) -> (x-y=w1791:dbl)
            n1169 = Square(x=w1790) -> (x^2=w1788:dbl)
            n1170 = Square(x=w1791) -> (x^2=w1789:dbl)
            n1171 = Add(x=w1789, y=w1788) -> (x+y=w1787:dbl)
            n1172 = Square Root(x=w1787) -> (sqrt(x)=w1784:dbl)
            n1173 = property on="Initial delta (MHz)" class="DigNum (strict)"("Val(Sgnl)"=w1784) -> ()  [unwired: 2 in, 2 out]
            n1174 = local write "Trap Delta (MHz)"(w1784) -> ()
          }
          frame True {
          }
        }
      }
      event "manual raster set": Value Change {
        n1175 = event-data() -> ()  [unwired: 7 out]
        n1176 = flat-sequence {
          frame #0 {
            n1177 = Replace Array Subset(array=u32[] [0] ("Index Values"), new element="manual raster set", index=0) -> (w1811:u32[])
            n1178 = property on="Saved AOD Raster Scan Parameter Sets" class="Arr (strict)"("Index Values"=w1811) -> ()  [unwired: 2 in, 2 out]
          }
          frame #1 {
            n1179 = property on="Load parameters" class="Bool (strict)"("Val(Sgnl)"=TRUE ("Value (Signaling)")) -> ()  [unwired: 2 in, 2 out]
          }
        }
      }
      event "Round T1 X": Value Change {
        n1180 = event-data() -> ()  [unwired: 7 out]
        n1181 = local read "BD 1 Frequency 1 (MHz)"() -> (w1818:dbl)
        n1182 = Round To Nearest(number=w1818) -> (nearest integer value=w1817:dbl)
        n1183 = property on="BD 1 Frequency 1 (MHz)" class="DigNum (strict)"("Val(Sgnl)"=w1817) -> ()  [unwired: 2 in, 2 out]
      }
      event "Round T2 X": Value Change {
        n1184 = event-data() -> ()  [unwired: 7 out]
        n1185 = local read "BD 1 Frequency 2 (MHz)"() -> (w1820:dbl)
        n1186 = Round To Nearest(number=w1820) -> (nearest integer value=w1819:dbl)
        n1187 = property on="BD 1 Frequency 2 (MHz)" class="DigNum (strict)"("Val(Sgnl)"=w1819) -> ()  [unwired: 2 in, 2 out]
      }
      event "Stop All": Value Change {
        n1188 = event-data() -> ()  [unwired: 7 out]
        n1189 = flat-sequence {
          tunnel: [w1826] -> w1824
          tunnel: [w1829] -> w1822
          tunnel: w1824 -> [w1829]
          tunnel: [TRUE] -> w1823
          frame #0 {
            n1190 = local read "Visa resource for valves"() -> (w1825:refnum<visa-resource-name>)
            n1191 = call "hamilton_controller.vi"("VISA resource name in"=w1825, "action"=T41."DISCONNECT") -> ("error out"=w1826:errorcluster)  [unwired: 8 in, 1 out]
          }
          frame #1 {
          }
        }
      }
      event "Delayed Interlace Start": Value Change {
        n1192 = event-data() -> ()  [unwired: 7 out]
        n1193 = flat-sequence {
          frame #0 {
            n1194 = Multiply(x="Delay to Interlace (s)", y=1000.0) -> (x*y=w1831:dbl)
            n1195 = Wait (ms)(milliseconds to wait=w1831) -> ()  [unwired: 1 out]
          }
          frame #1 {
            n1196 = property on="Laser interlacing mode" class="RadioBtnsControl (strict)"("Val(Sgnl)"=enum32{"Laser ON", "Laser OFF", "Interlace"}."Interlace" ("Value (Signaling)")) -> ()  [unwired: 2 in, 2 out]
          }
        }
      }
      event "BD 1 Amplitude 1 (%)", "BD 1 Amplitude 2 (%)", "BD 1 Amplitude 3 (%)", "BD 2 Amplitude 1 (%)", "BD 2 Amplitude 2 (%)", "BD 2 Amplitude 3 (%)", "Trap 1 ON", "Trap 2 ON", "Trap 3 ON", "Feedback On/Off", "All FB On/Off": Value Change {
        w1856 = i16 1 ("f")
        n1197 = event-data() -> ()  [unwired: 7 out]
        n1198 = local write "Trap 1 (ON/OFF)"("Trap 1 ON") -> ()
        n1199 = local write "Trap 2 (ON/OFF)"("Trap 2 ON") -> ()
        n1200 = Boolean To (0,1)(Boolean="Trap 3 ON") -> (0, 1=w1857:i16)
        n1201 = Boolean To (0,1)(Boolean="Trap 1 ON") -> (0, 1=w1858:i16)
        n1202 = Boolean To (0,1)(Boolean="Trap 2 ON") -> (0, 1=w1859:i16)
        n1203 = Select(t=w1859, s="Trap ON/OFF X or Y Amp?", f=w1856) -> (s? t:f=w1854:i16)
        n1204 = Select(t=w1858, s="Trap ON/OFF X or Y Amp?", f=w1856) -> (s? t:f=w1855:i16)
        n1205 = Select(t=w1857, s="Trap ON/OFF X or Y Amp?", f=w1856) -> (s? t:f=w1853:i16)
        n1206 = Select(t=w1856, s="Trap ON/OFF X or Y Amp?", f=w1859) -> (s? t:f=w1851:i16)
        n1207 = Select(t=w1856, s="Trap ON/OFF X or Y Amp?", f=w1858) -> (s? t:f=w1852:i16)
        n1208 = Select(t=w1856, s="Trap ON/OFF X or Y Amp?", f=w1857) -> (s? t:f=w1850:i16)
        n1209 = And(x="All FB On/Off", y="Feedback On/Off") -> (x .and. y?=w1848:cluster{"Set 1":bool, "Set 2":bool})
        n1210 = local read "BD 1 Amplitude 1 (%)"() -> (w1866:dbl)
        n1211 = local read "BD 1 Amplitude 2 (%)"() -> (w1865:dbl)
        n1212 = local read "BD 1 Amplitude 3 (%)"() -> (w1864:dbl)
        n1213 = Unbundle By Name(w1848) -> ("Set 1"=w1843:bool, "Set 2"=w1840:bool)
        n1214 = local read "Y RF Amplitude Limits (%)"() -> (w1836:T23)
        n1215 = local read "X RF Amplitude Limits (%)"() -> (w1837:T23)
        n1216 = local read "BD 2 Amplitude 1 (%)"() -> (w1867:dbl)
        n1217 = local read "BD 2 Amplitude 2 (%)"() -> (w1868:dbl)
        n1218 = local read "BD 2 Amplitude 3 (%)"() -> (w1869:dbl)
        n1219 = And(x="Trap 2 ON", y=w1840) -> (x .and. y?=w1838:bool)
        n1220 = And(x="Trap 1 ON", y=w1843) -> (x .and. y?=w1841:bool)
        n1221 = Multiply(x=w1855, y=w1866) -> (x*y=w1863:dbl)
        n1222 = Multiply(x=w1865, y=w1854) -> (x*y=w1861:dbl)
        n1223 = Multiply(x=w1864, y=w1853) -> (x*y=w1862:dbl)
        n1224 = Multiply(x=w1867, y=w1852) -> (x*y=w1870:dbl)
        n1225 = Multiply(x=w1868, y=w1851) -> (x*y=w1871:dbl)
        n1226 = Multiply(x=w1869, y=w1850) -> (x*y=w1872:dbl)
        n1227 = call "set RF board amplitude - interlace.vi"("Board 2 Amplitude Limits"=w1836, "Board 1 Amplitude Limits"=w1837, "FPGA VI Reference In"=w1835, "Board 2 Amplitude 3 (%)"=w1872, "Board 1 Amplitude 3 (%)"=w1862, "Board 2 Amplitude 2 (%)"=w1871, "Board 2 Amplitude 1 (%)"=w1870, "Board 1 Amplitude 2 (%)"=w1861, "Board 1 Amplitude 1 (%)"=w1863) -> ("error out"=w1845:errorcluster, "FPGA VI Reference Out"=w1846:T35)  [unwired: 1 in]
        n1228 = xnode "Read/Write Control"("FPGA VI Reference In"=w1846, "error in"=w1845, "FB On/Off Set 1"=w1841, "FB On/Off Set 2"=w1838) -> ("error out"=w1844:errorcluster)  [unwired: 1 out]
      }
      event "Load parameters": Value Change {
        n1229 = event-data() -> ()  [unwired: 7 out]
        n1230 = property on="Saved AOD Raster Scan Parameter Sets" class="Arr (strict)"() -> ("Index Values"=w1883:u32[])  [unwired: 2 in, 2 out]
        n1231 = Index Array(array=w1883, index=0) -> (element=w1880:u32)
        n1232 = local write "Load parameters"(FALSE ("Load parameters")) -> ()
        n1233 = Index Array(array="Saved AOD Raster Scan Parameter Sets", index=w1880) -> (element=w1879:T45)
        n1234 = Unbundle By Name(w1879) -> ("Scan Range AOD (nm) 2"=w1878:dbl, "Step Size AOD (nm) 2"=w1877:dbl, "Scan Speed AOD (nm/s) 2"=w1876:dbl, "Number of scans (AOD) 2"=w1875:u16)
        n1235 = flat-sequence {
          tunnel: w1878 -> [w1886]
          tunnel: w1877 -> [w1885]
          tunnel: w1876 -> [w1884]
          tunnel: w1875 -> [w1887]
          frame #0 {
            n1236 = local write "Scan Speed (nm/s)"(w1884) -> ()
            n1237 = local write "Scan Range (nm)"(w1886) -> ()
            n1238 = local write "Step Size (nm)"(w1885) -> ()
          }
          frame #1 {
            n1239 = property on="Number of F/B Scans (AOD)" class="DigNum (strict)"("Val(Sgnl)"=w1887) -> ()  [unwired: 2 in, 2 out]
          }
        }
      }
      event "Trap 1 (ON/OFF)", "Trap 2 (ON/OFF)": Value Change {
        n1240 = event-data() -> ()  [unwired: 7 out]
        n1241 = flat-sequence {
          tunnel: [w1897] -> w1892
          tunnel: w1892 -> [w1912]
          tunnel: [w1898] -> w1888
          frame #0 {
            n1242 = local read "Trap 1 ON"() -> (w1897:bool)
          }
          frame #1 {
            n1243 = Exclusive Or(1:w1912, 2:"Trap 1 (ON/OFF)") -> (0:w1905:bool)
            n1244 = Select(t="on", s="Trap 2 (ON/OFF)", f="off") -> (s? t:f=w1904:string)
            n1245 = Select(t="on", s="Trap 1 (ON/OFF)", f="off") -> (s? t:f=w1900:string)
            n1246 = Build Array("trap 1 ", w1900) -> (w1899:string[])
            n1247 = Build Array("trap 2 " ("f"), w1904) -> (w1902:string[])
            n1248 = Select(t=w1899, s=w1905, f=w1902) -> (s? t:f=w1898:string[])
            n1249 = property on="Trap 1 ON" class="Bool (strict)"("Val(Sgnl)"="Trap 1 (ON/OFF)") -> ()  [unwired: 2 in, 2 out]
            n1250 = property on="Trap 2 ON" class="Bool (strict)"("Val(Sgnl)"="Trap 2 (ON/OFF)") -> ()  [unwired: 2 in, 2 out]
          }
        }
        n1251 = local read "Saving..."() -> (w1891:bool)
        n1252 = local read "Save Event Log?"() -> (w1890:bool)
        n1253 = And(x=w1891, y=w1890) -> (x .and. y?=w1889:bool)
        n1254 = case shown="True" w1889 {
          tunnel: w1888 -> [_ w1896]
          frame False {
          }
          frame True {
            n1255 = local read "Time (s)"() -> (w1893:dbl)
            n1256 = local read "log file ref"() -> (w1895:refnum<file>)
            n1257 = Concatenate Strings(w1896) -> (w1894:string)
            n1258 = call "write to event log.vi"("log file ref"=w1895, "time"=w1893, "input string"=w1894) -> ()  [unwired: 8 in]
          }
        }
      }
      event "DIO count 1 (ticks)", "DIO count 2 (ticks)", "DIO count 3 (ticks)", "Interlace", "Number Interlace Sets", "Not-Interlacing Set", "BD 1 Delay (ticks)", "BD 2 Delay (Ticks)", "Next trap write delay (ticks)", "XY phase ext loop method", "Amp switch delay 2", "BD 2 Delay (Ticks) 2", "BD 1 Delay (ticks) 2": Value Change {
        n1259 = event-data() -> ()  [unwired: 7 out]
        n1260 = To Unsigned Byte Integer(number="Not-Interlacing Set") -> (unsigned 8bit integer=w1913:u8)
        n1261 = Add(x=u8 1 ("y"), y=w1913) -> (x+y=w1922:u8)
        n1262 = local read "DIO count 1 (ticks)"() -> (w1929:u16)
        n1263 = local read "DIO count 2 (ticks)"() -> (w1928:u16)
        n1264 = local read "DIO count 3 (ticks)"() -> (w1927:u16)
        n1265 = xnode "Read/Write Control"("FPGA VI Reference In"=w1915, "DIO count 1 (ticks)"=w1929, "DIO count 2 (ticks)"=w1928, "DIO count 3 (ticks)"=w1927, "Interlace ON/OFF"="Interlace", "Number Interlace Cycles"="Number Interlace Sets", "Interlace Off Parameters"=w1922, "BD 1 Delay (ticks)"="BD 1 Delay (ticks)", "BD 2 Delay (Ticks)"="BD 2 Delay (Ticks)", "Next trap write delay (ticks)"="Next trap write delay (ticks)") -> ("error out"=w1931:errorcluster)  [unwired: 1 in, 1 out]
        n1266 = Build Array(w1929, w1928, w1927) -> (w1921:u16[])
        n1267 = Split 1D Array(array=w1921, index="Number Interlace Sets") -> (first subarray=w1930:u16[])  [unwired: 1 out]
        n1268 = Index Array(array=w1921, index=w1913) -> (element=w1920:u16)
        n1269 = Add Array Elements(numeric array=w1930) -> (sum=w1924:u16)
        n1270 = Select(t=w1924, s="Interlace", f=w1920) -> (s? t:f=→"Total Counts (ticks)":u16)
      }
      event "Reset Feedback": Value Change {
        n1271 = event-data() -> ()  [unwired: 7 out]
        n1272 = Unbundle By Name("Reset Feedback") -> ("Set 1"=w1935:bool, "Set 2"=w1934:bool)
        n1273 = xnode "Read/Write Control"("FPGA VI Reference In"=w1932, "FB Reset Set 1"=w1935, "FB Reset Set 2"=w1934) -> ("error out"=w1933:errorcluster)  [unwired: 1 in, 1 out]
      }
      event "Trap intensity output range", "Trap Intensity PID Gains": Value Change {
        n1274 = event-data() -> ()  [unwired: 7 out]
        n1275 = xnode "Read/Write Control"("FPGA VI Reference In"=w1939, "FB Gains"="Trap Intensity PID Gains", "FB output range"="Trap intensity output range") -> ("error out"=w1940:errorcluster)  [unwired: 1 in, 1 out]
      }
      event "AI2 to Setpoint", "Setpoints (V)": Value Change {
        n1276 = event-data() -> ()  [unwired: 7 out]
        n1277 = xnode "Read/Write Control"("FPGA VI Reference In"=w1941) -> ("FPGA VI Reference Out"=w1944:T35, "error out"=w1943:errorcluster, "AI2 Y Sum Set 1"=w1951:i16, "AI2 Y Sum Set 2"=w1950:i16)  [unwired: 1 in]
        n1278 = Cluster To Array(cluster="AI2 to Setpoint") -> (array=w1954:bool[])
        n1279 = local read "AI2 (V)"() -> (w1952:cluster{"Set 1":dbl, "Set 2":dbl})
        n1280 = Or Array Elements(Boolean array=w1954) -> (logical OR=w1955:bool)
        n1281 = Bundle By Name(cluster=w1952, "Set 1"=w1951, "Set 2"=w1950) -> (w1949:cluster{"Set 1":dbl, "Set 2":dbl})
        n1282 = Divide(x=w1949, y=3276.7) -> (x/y=w1948:cluster{"Set 1":dbl, "Set 2":dbl})
        "AI2 (V)" <- w1948
        n1283 = case shown="True" w1955 {
          tunnel: [w1958 w1975] -> w1947
          tunnel: "AI2 to Setpoint" -> [_ w1971]
          tunnel: "Setpoints (V)" -> [w1959 w1974]
          tunnel: w1948 -> [_ w1968]
          frame False {
            n1284 = Multiply(x=3276.7, y=w1959) -> (x*y=w1960:cluster{"Set 1":dbl, "Set 2":dbl})
            n1285 = To Word Integer(number=w1960) -> (16bit integer=w1958:cluster{"Set 1":i16, "Set 2":i16})
          }
          frame True {
            n1286 = Unbundle By Name(w1968) -> ("Set 1"=w1967:dbl, "Set 2"=w1966:dbl)
            n1287 = Unbundle By Name(w1974) -> ("Set 1"=w1973:dbl, "Set 2"=w1972:dbl)
            n1288 = Unbundle By Name(w1971) -> ("Set 1"=w1970:bool, "Set 2"=w1969:bool)
            n1289 = Select(t=w1967, s=w1970, f=w1973) -> (s? t:f=w1965:dbl)
            n1290 = Select(t=w1966, s=w1969, f=w1972) -> (s? t:f=w1964:dbl)
            n1291 = Bundle By Name(cluster=w1974, "Set 1"=w1965, "Set 2"=w1964) -> (w1962:cluster{"Set 1":dbl, "Set 2":dbl})
            n1292 = local write "Setpoints (V)"(w1962) -> ()
            n1293 = Multiply(x=3276.7, y=w1962) -> (x*y=w1963:cluster{"Set 1":dbl, "Set 2":dbl})
            n1294 = To Word Integer(number=w1963) -> (16bit integer=w1975:cluster{"Set 1":i16, "Set 2":i16})
          }
        }
        n1295 = Unbundle By Name(w1947) -> ("Set 1"=w1946:i16, "Set 2"=w1945:i16)
        n1296 = xnode "Read/Write Control"("FPGA VI Reference In"=w1944, "error in"=w1943, "FB Setpoint Set 1"=w1946, "FB Setpoint Set 2"=w1945) -> ("error out"=w1942:errorcluster)  [unwired: 1 out]
      }
      event "+ phase (GI)", "- phase (GI)", "+ phase (GI) 2", "- phase (GI) 2", "+ phase (RI)", "- phase (RI)", "+ phase (Green FB)", "- phase (Green FB)", "- phase (BI AO)", "+ phase (BI AO)", "- phase (BI DO)", "+ phase (BI DO)": Value Change {
        n1297 = event-data() -> ()  [unwired: 7 out]
        n1298 = Or(x="+ phase (GI)", y="- phase (GI)") -> (x .or. y?=w2011:bool)
        n1299 = Negate(x="Phase adj. (GI)") -> (-x=w2016:i16)
        n1300 = Select(t=w2016, s="+ phase (GI)", f="Phase adj. (GI)") -> (s? t:f=w2015:i16)
        n1301 = Or(x="+ phase (GI) 2", y="- phase (GI) 2") -> (x .or. y?=w2002:bool)
        n1302 = Negate(x="Phase adj. (GI) 2") -> (-x=w2007:i16)
        n1303 = Select(t=w2007, s="+ phase (GI) 2", f="Phase adj. (GI) 2") -> (s? t:f=w2003:i16)
        n1304 = Negate(x="Phase adj. (RI)") -> (-x=w2001:i16)
        n1305 = Or(x="+ phase (RI)", y="- phase (RI)") -> (x .or. y?=w1997:bool)
        n1306 = Select(t=w2001, s="+ phase (RI)", f="Phase adj. (RI)") -> (s? t:f=w1996:i16)
        n1307 = Or(x="+ phase (Green FB)", y="- phase (Green FB)") -> (x .or. y?=w1990:bool)
        n1308 = Negate(x="Phase adj. (Green FB)") -> (-x=w1995:i16)
        n1309 = Select(t=w1995, s="+ phase (Green FB)", f="Phase adj. (Green FB)") -> (s? t:f=w1991:i16)
        n1310 = Negate(x="Phase adj. (BI AO)") -> (-x=w1989:i16)
        n1311 = Or(x="+ phase (BI AO)", y="- phase (BI AO)") -> (x .or. y?=w1979:bool)
        n1312 = Select(t=w1989, s="+ phase (BI AO)", f="Phase adj. (BI AO)") -> (s? t:f=w1981:i16)
        n1313 = Negate(x="Phase adj. (BI DO)") -> (-x=w1985:i16)
        n1314 = Or(x="+ phase (BI DO)", y="- phase (BI DO)") -> (x .or. y?=w1978:bool)
        n1315 = Select(t=w1985, s="+ phase (BI DO)", f="Phase adj. (BI DO)") -> (s? t:f=w1980:i16)
        n1316 = xnode "Read/Write Control"("FPGA VI Reference In"=w1977, "Phase count adjustment (GI)"=w2015, "Phase count adjustment (GI) 2"=w2003, "Phase count adjustment (RI)"=w1996, "Phase count adjustment (Green FB)"=w1991, "Phase count adjustment (BI AO)"=w1981, "Phase count adjustment (BI D)"=w1980) -> ("FPGA VI Reference Out"=w2013:T35, "error out"=w2014:errorcluster)  [unwired: 1 in]
        n1317 = xnode "Read/Write Control"("FPGA VI Reference In"=w2013, "error in"=w2014, "+ phase (GI)"=w2011, "+ phase (GI) 2"=w2002, "+ phase (RI)"=w1997, "+ phase (Green FB)"=w1990, "+ phase (BI AO)"=w1979, "+ phase (BI D)"=w1978) -> ("error out"=w2012:errorcluster)  [unwired: 1 out]
      }
      event "Green Laser ON/OFF", "Red Laser ON/OFF", "Blue Laser ON/OFF": Value Change {
        # "This loop shouldn't be initialized.  The main 'laser ON' settings should dominate and set the others."
        n1318 = event-data() -> ()  [unwired: 7 out]
        n1319 = property on="Red Laser ON" class="Bool (strict)"("Val(Sgnl)"="Red Laser ON/OFF") -> ()  [unwired: 2 in, 2 out]
